vi "Button and Menu Status.vi"(11 "Target List":i32[](array[numeric])) -> (2 "View Target Info":bool, 3 "Configure Target":bool)   [LabVIEW 2020]
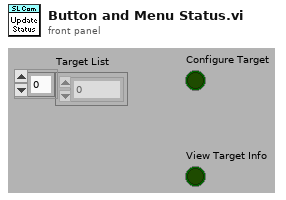
[diagram p1: front panel]
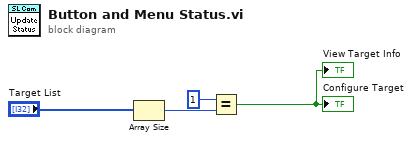
[diagram p0: block diagram]
diagram:
  n1 = Array Size(array="Target List") -> (size(s)=w3:i32)
  n2 = Equal?(x=1, y=w3) -> (x = y?=→"Configure Target" →"View Target Info":bool)
